vi "test-PID-test-00-InitialSettings.vi"() -> (3 "All Passed":bool)   [LabVIEW 2019]
uses:
  <vilib>/Rock Robotics/WPI/ThirdParty/JAS_Junk/TrajLib/Trajectory_Library.lvlib
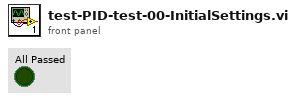
[diagram p1: front panel]
types:
  T1 = typedef "Trajectory_Library.lvlib/PID_CONTROLLER.ctl" = cluster{"Kp":dbl, "Ki":dbl, "Kd":dbl, "Period":dbl, "Max_Integral":dbl, "Min_Integral":dbl, "Max_Input":dbl, "Min_Input":dbl, "Continuous":bool, "PositionError":dbl, "VelocityError":dbl, "PrevError":dbl, "TotalError":dbl, "PositionTolerance":dbl, "VelocityTolerance":dbl, "SetPoint":dbl, "Kf":dbl, "Prev_Deriv":dbl, "Prev_Deriv 2":dbl, "DerivativeFilter":bool, "Min_Output":dbl, "Max_Output":dbl, "Prev_F_P":dbl, "Prev_F_P_2":dbl, "AntiWindupActive":bool, "Measurement":dbl}
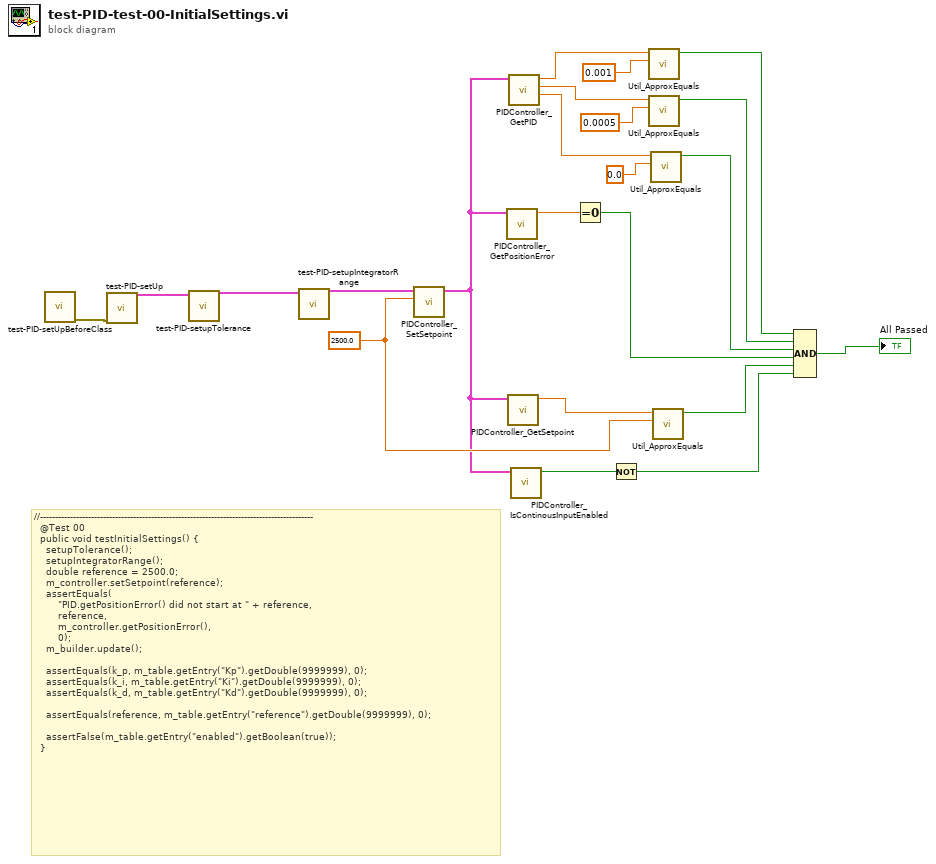
[diagram p0: block diagram]
diagram:
  w5 = 2500.0 ("Setpoint")
  # "//-------------------------------------------------------------------------------------------\n  @Test 00\n  public void testInitialSettings() {\n    setupTolerance();\n    setupIntegratorRange();\n    double reference = 2500.0;\n    m_controller.setSetpoint(reference);\n    assertEquals(\n        \"PID.getPositionError() did not start at \" + reference,\n        reference,\n        m_controller.getPositionError(),\n        0);\n    m_builder.update();\n\n    assertEquals(k_p, m_table.getEntry(\"Kp\").getDouble(9999999), 0);\n    assertEquals(k_i, m_table.getEntry(\"Ki\").getDouble(9999999), 0);\n    assertEquals(k_d, m_table.getEntry(\"Kd\").getDouble(9999999), 0);\n\n    assertEquals(reference, m_table.getEntry(\"reference\").getDouble(9999999), 0);\n\n    assertFalse(m_table.getEntry(\"enabled\").getBoolean(true));\n  }"
  n1 = call "test-PID-setUpBeforeClass.vi"() -> ("error out"=w21:errorcluster)  [unwired: 11 in]
  n2 = call "test-PID-setUp.vi"("error in (no error)"=w21) -> ("PID_CONTROLLER"=w20:T1)  [unwired: 9 in, 1 out]
  n3 = call "test-PID-setupTolerance.vi"("in PID_CONTROLLER"=w20) -> ("out PID_CONTROLLER"=w19:T1)  [unwired: 10 in]
  n4 = call "test-PID-setupIntegratorRange.vi"("in PID_CONTROLLER"=w19) -> ("out PID_CONTROLLER"=w18:T1)  [unwired: 10 in]
  n5 = call <vilib>:"PIDController_SetSetpoint.vi"("Setpoint"=w5, "in PID_CONTROLLER"=w18) -> ("out PID_CONTROLLER"=w3:T1)  [unwired: 9 in]
  n6 = call <vilib>:"PIDController_GetPositionError.vi"("in PID_CONTROLLER"=w3) -> ("PositionError"=w17:dbl)  [unwired: 10 in]
  n7 = call <vilib>:"PIDController_GetSetpoint.vi"("in PID_CONTROLLER"=w3) -> ("Setpoint"=w6:dbl)  [unwired: 10 in]
  n8 = call <vilib>:"PIDController_GetPID.vi"("in PID_CONTROLLER"=w3) -> ("Kd"=w11:dbl, "Ki"=w13:dbl, "Kp"=w15:dbl)  [unwired: 8 in]
  n9 = call <vilib>:"PIDController_IsContinousInputEnabled.vi"("in PID_CONTROLLER"=w3) -> ("ContinousInputEnabled"=w2:bool)  [unwired: 10 in]
  n10 = Equal To 0?(x=w17) -> (x = 0?=w16:bool)
  n11 = Not(x=w2) -> (.not. x?=w1:bool)
  n12 = call <vilib>:"Util_ApproxEquals.vi"("Value 2"=0.001, "Value 1"=w15) -> ("ApproxEquals"=w7:bool)  [unwired: 9 in]
  n13 = call <vilib>:"Util_ApproxEquals.vi"("Value 2"=0.0005, "Value 1"=w13) -> ("ApproxEquals"=w8:bool)  [unwired: 9 in]
  n14 = call <vilib>:"Util_ApproxEquals.vi"("Value 2"=0.0, "Value 1"=w11) -> ("ApproxEquals"=w9:bool)  [unwired: 9 in]
  n15 = call <vilib>:"Util_ApproxEquals.vi"("Value 2"=w5, "Value 1"=w6) -> ("ApproxEquals"=w4:bool)  [unwired: 9 in]
  n16 = Compound Arithmetic op=AND(w7, w8, w9, w16, w4, w1) -> (→"All Passed":bool)
